vi "write.vi"(1 "Infos":u8[](array[numeric])) -> (0 "to write":string)   [LabVIEW 2022 SP3]
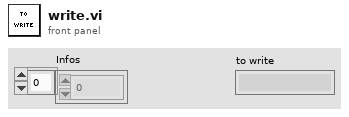
[diagram p1: front panel]
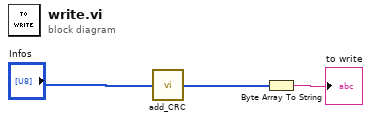
[diagram p0: block diagram]
diagram:
  n1 = call "add_CRC.vi"("Raw Data"="Infos") -> ("Data + CRC"=w1:u8[])
  n2 = Byte Array To String(unsigned byte array=w1) -> (string=→"to write":string)
